vi "Teleop - Climb Safety (SubVI).vi"(7 "Desired cluster In":T1 {"shooterMotorMode" items=["PercentOutput"=0, "Position"=1, "Velocity"=2, "Current"=3, "Follower"=5, "MotionProfile"=6, "MotionMagic"=7, "MotionProfileArc"=10, "Disabled"=15]}, 12 "Climb":bool) -> (8 "Desired cluster out":T1 {"shooterMotorMode" items=["PercentOutput"=0, "Position"=1, "Velocity"=2, "Current"=3, "Follower"=5, "MotionProfile"=6, "MotionMagic"=7, "MotionProfileArc"=10, "Disabled"=15]})   [LabVIEW 2019]
uses:
  Desired Cluster.ctl
  <vilib>/Rock Robotics/WPI/ThirdParty/Phoenix-LabVIEW/Motor Controller/Controls/CTRE_Phoenix_MotorControl_ControlMode.ctl
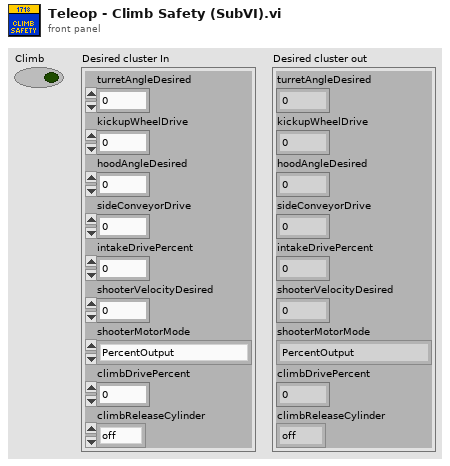
[diagram p1: front panel]
types:
  T1 = typedef "Desired Cluster.ctl" = cluster{"turretAngleDesired":dbl, "kickupWheelDrive":dbl, "hoodAngleDesired":dbl, "sideConveyorDrive":dbl, "intakeDrivePercent":dbl, "shooterVelocityDesired":dbl, "shooterMotorMode":T2, "climbDrivePercent":dbl, "climbReleaseCylinder":enum16{"off", "on", "forward", "back"}}
  T2 = typedef "CTRE_Phoenix_MotorControl_ControlMode.ctl" = u16
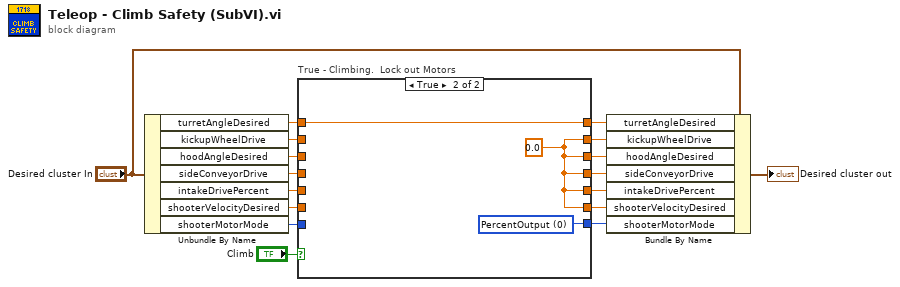
[diagram p0: block diagram]
diagram:
  n1 = Unbundle By Name("Desired cluster In") -> ("turretAngleDesired"=w16:dbl, "kickupWheelDrive"=w15:dbl, "hoodAngleDesired"=w14:dbl, "sideConveyorDrive"=w13:dbl, "intakeDrivePercent"=w12:dbl, "shooterVelocityDesired"=w11:dbl, "shooterMotorMode"=w10:T2)
  n2 = case "True - Climbing.  Lock out Motors" shown="True" "Climb" {
    tunnel: w16 -> [w24 w27]
    tunnel: [w24 w27] -> w7
    tunnel: w15 -> [w23 _]
    tunnel: [w23 w26] -> w6
    tunnel: [w22 w26] -> w5
    tunnel: w14 -> [w22 _]
    tunnel: [w21 w26] -> w4
    tunnel: w13 -> [w21 _]
    tunnel: [w20 w26] -> w3
    tunnel: w12 -> [w20 _]
    tunnel: w11 -> [w18 _]
    tunnel: w10 -> [w19 _]
    tunnel: [w18 w26] -> w2
    tunnel: [w19 w25] -> w1
    frame False {
    }
    frame True {
      w25 = T2 0 items=["PercentOutput"=0, "Position"=1, "Velocity"=2, "Current"=3, "Follower"=5, "MotionProfile"=6, "MotionMagic"=7, "MotionProfileArc"=10, "Disabled"=15] ("shooterMotorMode")
      w26 = 0.0 ("turretAngleManualPosition")
    }
  }
  n3 = Bundle By Name(cluster="Desired cluster In", "turretAngleDesired"=w7, "kickupWheelDrive"=w6, "hoodAngleDesired"=w5, "sideConveyorDrive"=w4, "intakeDrivePercent"=w3, "shooterVelocityDesired"=w2, "shooterMotorMode"=w1) -> (→"Desired cluster out":T1)
